vi "Xml_GetValueByName.vi"(8 "offset (0)":i32, 9 "TagName":string, 11 "XML String":string) -> (2 "offset past match":i32, 3 "TagValue":string)   [LabVIEW 2021, in "XML.lvlib"]
uses:
  XML.lvlib
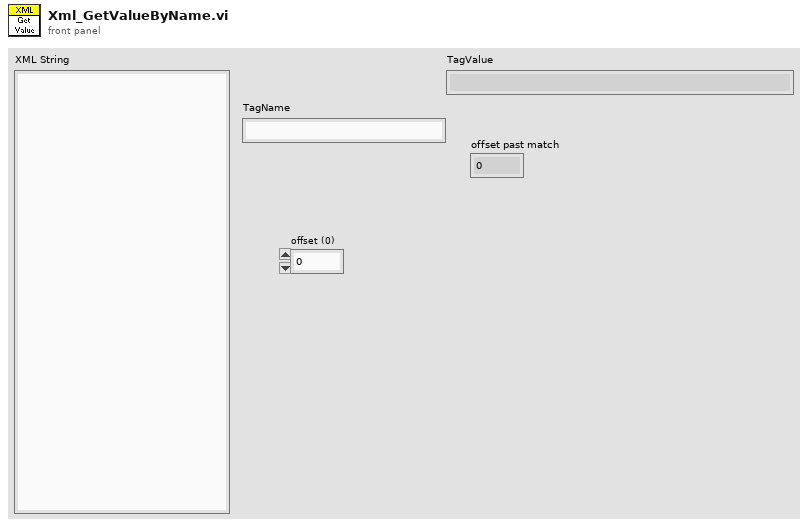
[diagram p1: front panel]
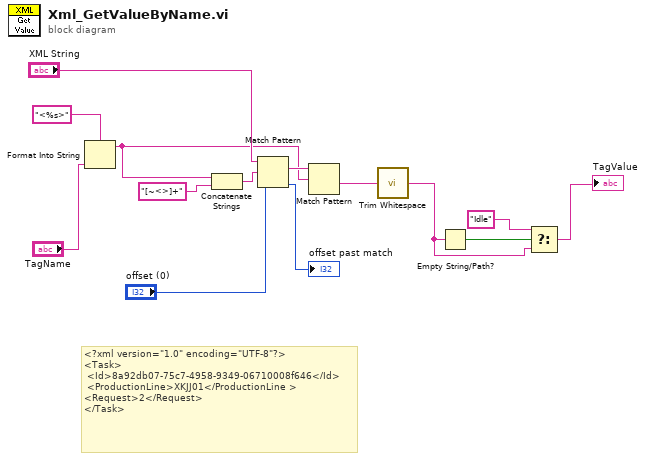
[diagram p0: block diagram]
diagram:
  # "<?xml version=\"1.0\" encoding=\"UTF-8\"?>\n<Task>\n\t<Id>8a92db07-75c7-4958-9349-06710008f646</Id>\n\t<ProductionLine>XKJJ01</ProductionLine >\n<Request>2</Request>\n</Task>"
  n1 = Format Into String(format string="<%s>" ("regular expression"), "TagName") -> (resulting string=w3:string)  [unwired: 2 in, 1 out]
  n2 = Concatenate Strings(w3, "[~<>]+" ("string")) -> (w14:string)
  n3 = Match Pattern(string="XML String", regular expression=w14, offset (0)="offset (0)") -> (match substring=w12:string, offset past match=→"offset past match":i32)  [unwired: 2 out]
  n4 = Match Pattern(string=w12, regular expression=w3) -> (after substring=w10:string)  [unwired: 1 in, 3 out]
  n5 = call <vilib>:"Trim Whitespace.vi"("string"=w10) -> ("trimmed string"=w7:string)  [unwired: 1 in]
  n6 = Empty String/Path?(string/path=w7) -> (empty?=w8:bool)
  n7 = Select(t="Idle", s=w8, f=w7) -> (s? t:f=→"TagValue":string)
